vi "getFont.vi"(0 "reference":refnum<class "Graphics.lvclass">, 5 "error in (no error)":errorcluster) -> (14 "reference out":refnum<class "Graphics.lvclass">, 15 "fontType":T2=enum."Application Font", 16 "font":T1, 17 "size":i16, 19 "error out":errorcluster)   [LabVIEW 2016, in "Graphics.lvclass"]
doc: "Get font info"
uses:
  <resource>/Framework/Providers/Open_GDS/UML/Graphics_class/Graphics.lvclass
  <resource>/Framework/Providers/Open_GDS/UML/Graphics_class/LvFontType.ctl
  <resource>/Framework/Providers/Open_GDS/UML/Graphics_class/FontType.ctl
panel:
  # "Always set\nVI Server class\nto current VI. Do not\nconnect this control\nto the connector pane.\n(Tip!: Just drag\nand drop the icon\ninto the refnum)"
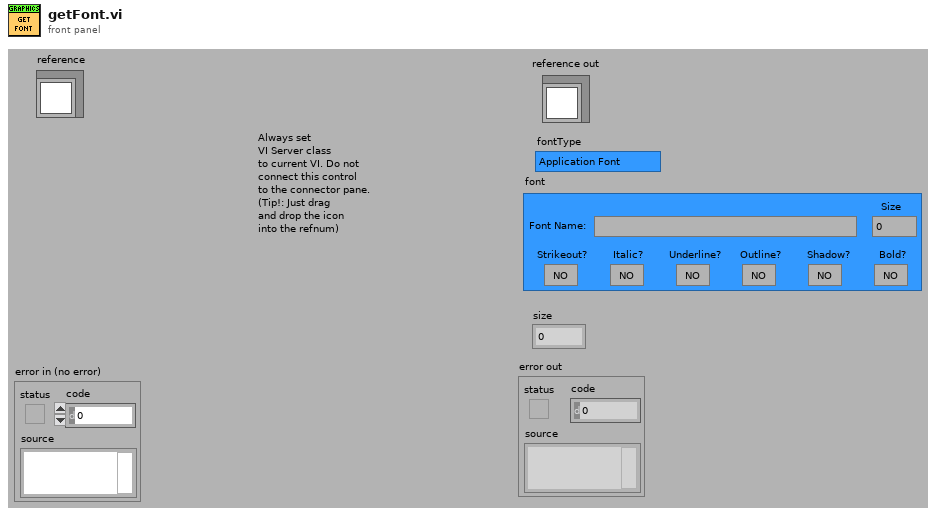
[diagram p1: front panel]
types:
  T1 = typedef "Graphics.lvclass/FontType.ctl" = cluster{"Font Name:":string, "Size":i16, "Strikeout?":bool, "Italic?":bool, "Underline?":bool, "Outline?":bool, "Shadow?":bool, "Bold?":bool}
  T2 = typedef "Graphics.lvclass/LvFontType.ctl" = enum16{"User-specified Font", "Application Font", "System Font", "Dialog Font"}
  T3 = typedef "Graphics.lvclass/ObjectAttributes.ctl" = cluster{"drawColor":u32, "backgroundColor":u32, "font":T1, "fontType":T2, "picture":picture, "stroke":T4, "scaleX":dbl, "scaleY":dbl, "screenRef":refnum<vi>, "offsetX":dbl, "offsetY":dbl}
  T4 = typedef "Graphics.lvclass/StrokeType.ctl" = enum16{"USE_DEFAULT", "SOLID", "DOTTED"}
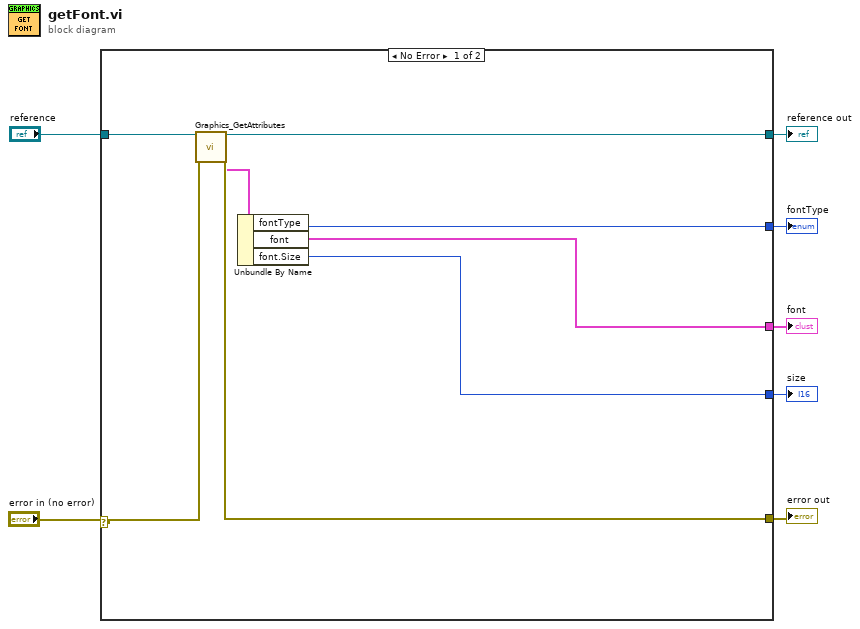
[diagram p0: block diagram]
diagram:
  n1 = case shown="No Error" "error in (no error)" {
    selector: "error in (no error)" -> [w9 w16]
    tunnel: "reference" -> [w15 w17]
    tunnel: [w14 w16] -> w6
    tunnel: [w13 w17] -> w5
    tunnel: [w12 _] -> w3
    tunnel: [w11 _] -> w2
    tunnel: [w10 _] -> w1
    frame No Error {
      n2 = call <resource>:"Graphics_GetAttributes.vi"("reference in"=w15, "error in (no error)"=w9) -> ("reference out"=w13:refnum<class "Graphics.lvclass">, "Data"=w8:T3, "error out"=w14:errorcluster)  [unwired: 1 in, 14 out]
      n3 = Unbundle By Name(w8) -> ("fontType"=w12:T2, "font"=w11:T1, "font.Size"=w10:i16)
    }
    frame Error {
    }
  }
  "reference out" <- w5
  "error out" <- w6
  "size" <- w1
  "font" <- w2
  "fontType" <- w3
